vi "validateNewBalls.vi"(7 "timeToValidateBall":dbl=0.5, 8 "error in (no error)":errorcluster, 10 "array of cameras in":T1[](array[typedef]) {"robots_blue"."height" format="%+4.3f"; "robots_blue"."pixel_y" format="%+4.3f"; "robots_blue"."pixel_x" format="%+4.3f"; "robots_blue"."orientation" format="%+4.3f"; "robots_blue"."y" format="%+4.3f"; "robots_blue"."confidence" format="%4.3f"; "robots_blue"."x" format="%+4.3f"; "robots_yellow"."height" format="%+4.3f"; "robots_yellow"."pixel_y" format="%+4.3f"; "robots_yellow"."pixel_x" format="%+4.3f"; "robots_yellow"."orientation" format="%+4.3f"; "robots_yellow"."y" format="%+4.3f"; "robots_yellow"."confidence" format="%4.3f"; "robots_yellow"."x" format="%+4.3f"}, 11 "Vision in":refnum<class "Vision.lvclass">) -> (0 "error out":errorcluster, 2 "Array of cameras out":T1[](array[typedef]) {"robots_blue"."height" format="%+4.3f"; "robots_blue"."pixel_y" format="%+4.3f"; "robots_blue"."pixel_x" format="%+4.3f"; "robots_blue"."orientation" format="%+4.3f"; "robots_blue"."y" format="%+4.3f"; "robots_blue"."confidence" format="%4.3f"; "robots_blue"."x" format="%+4.3f"; "robots_yellow"."height" format="%+4.3f"; "robots_yellow"."pixel_y" format="%+4.3f"; "robots_yellow"."pixel_x" format="%+4.3f"; "robots_yellow"."orientation" format="%+4.3f"; "robots_yellow"."y" format="%+4.3f"; "robots_yellow"."confidence" format="%4.3f"; "robots_yellow"."x" format="%+4.3f"}, 3 "Vision out":refnum<class "Vision.lvclass">)   [LabVIEW 2022 SP3, in "Vision.lvclass"]
uses:
  Vision.lvclass
  Old vision/Controls/SSL Detection Frame.ctl
  Old vision/Controls/SSL Detection Robot.ctl
  <vilib>/Analysis/Matrix/Datatypes/RealMatrix.ctl
  Old vision/Controls/SSL Detection Ball.ctl
  newBallValidate.ctl
  <vilib>/Analysis/_algsub.llb/Real Vector Norm.vi
  <vilib>/Analysis/NI_AALPro.lvlib
  <vilib>/Analysis/Matrix/NI_Matrix.lvlib
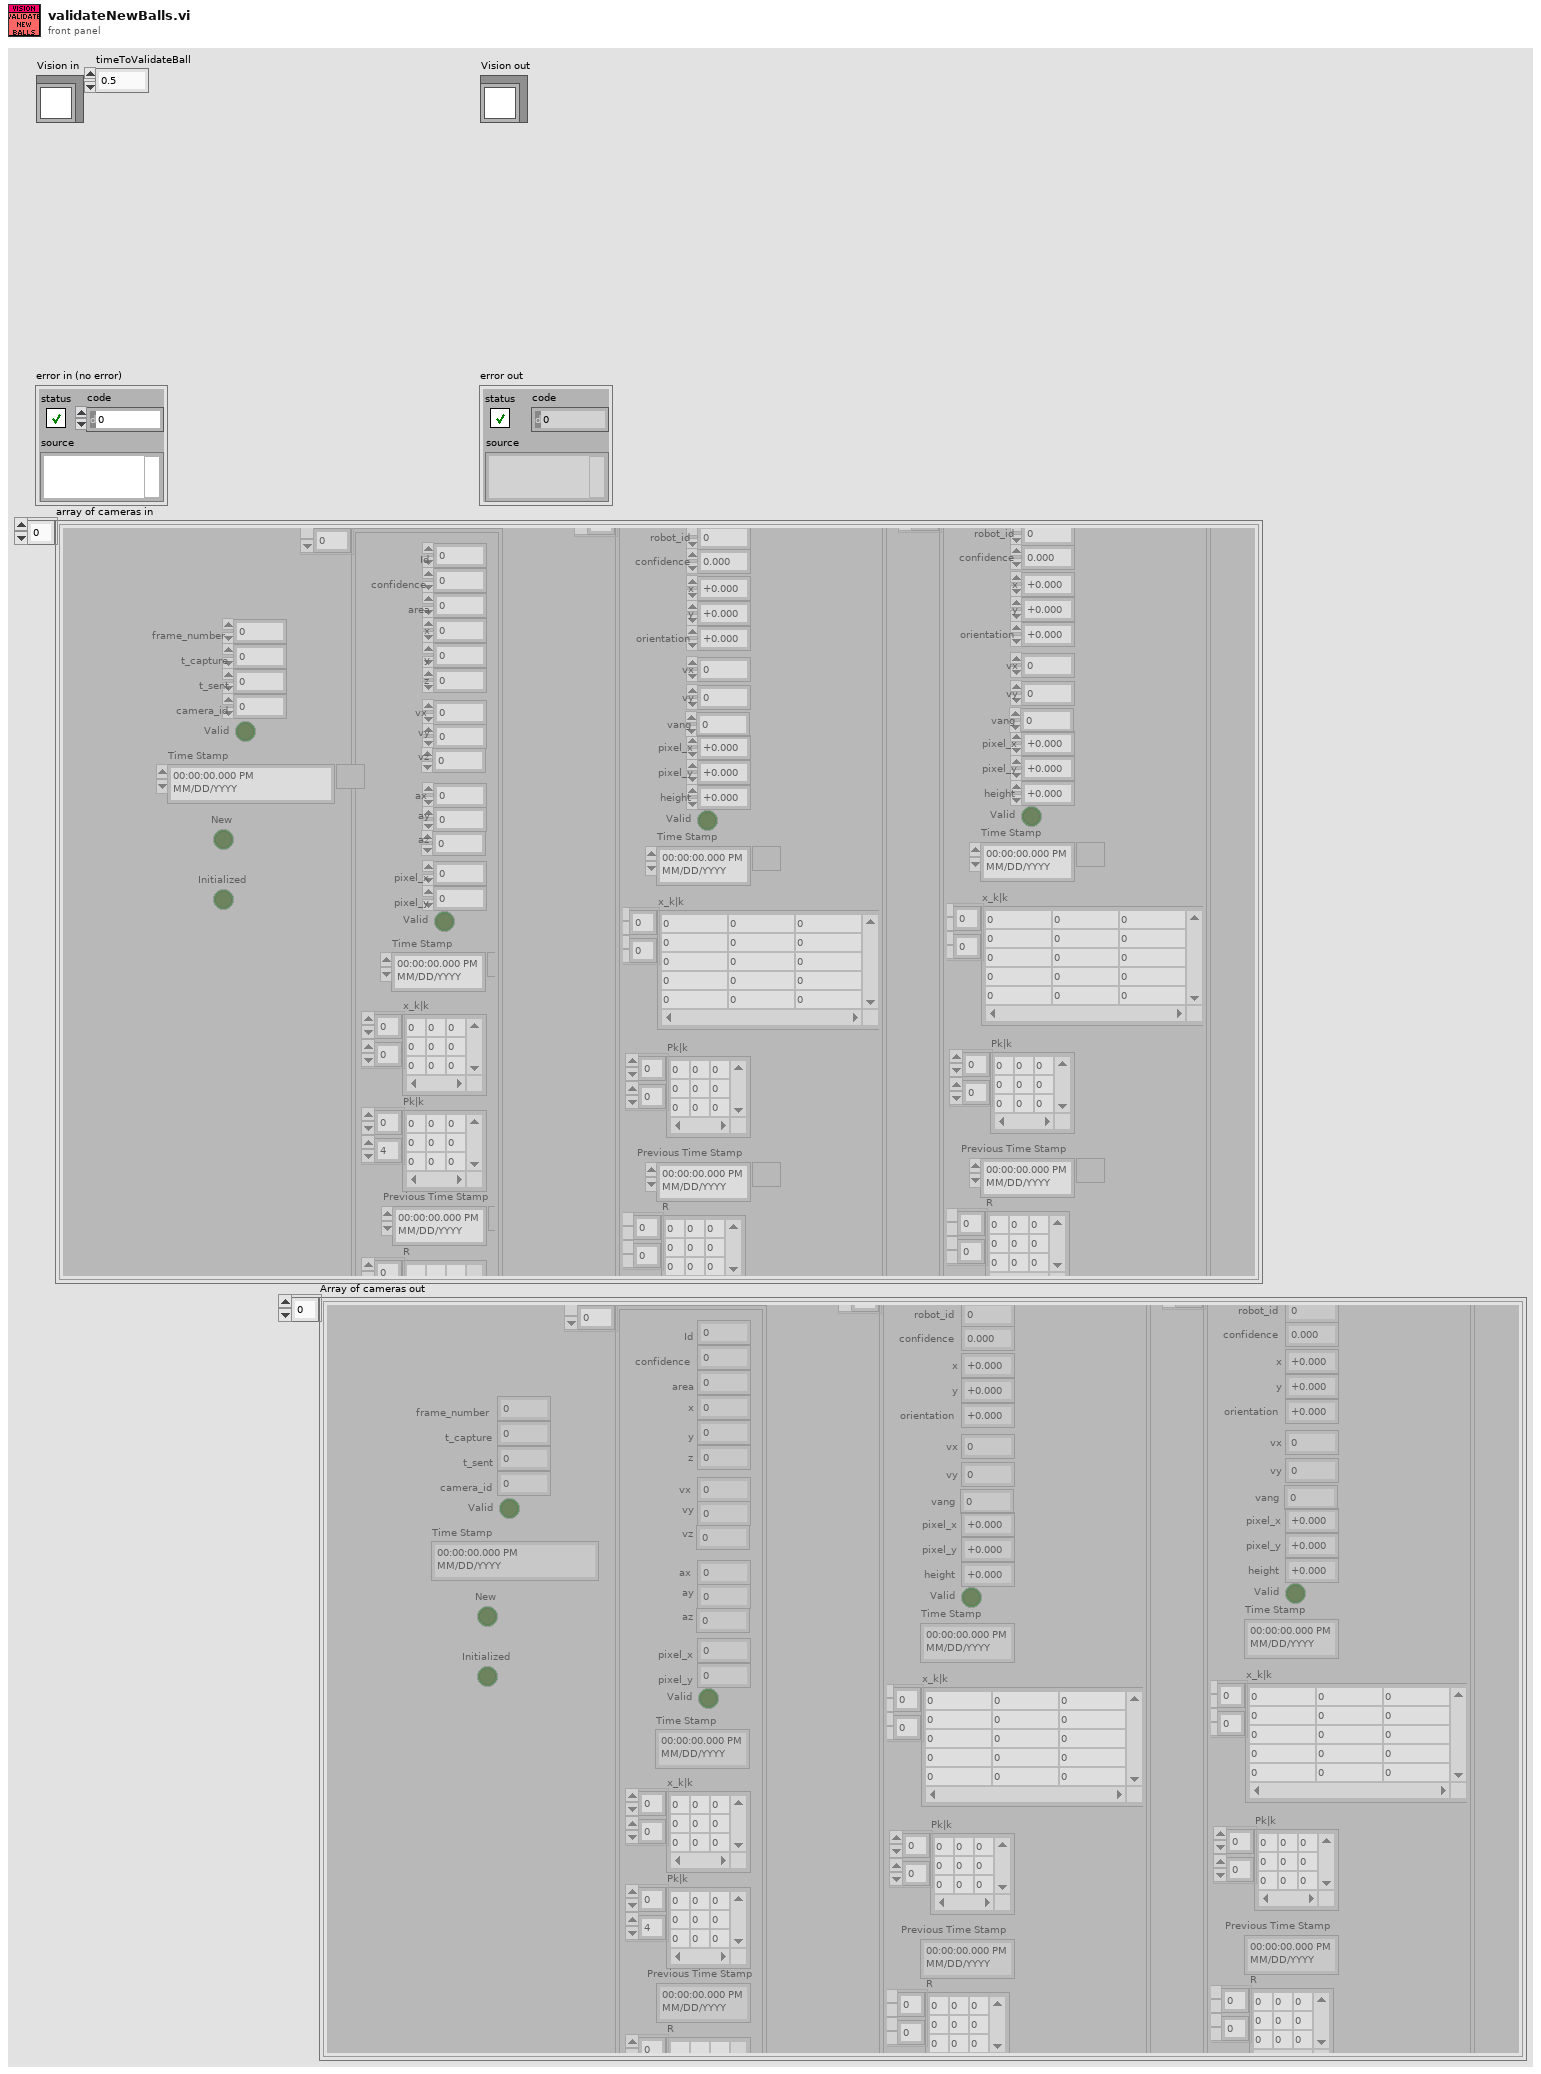
[diagram p1: front panel]
types:
  T1 = typedef "SSL Detection Frame.ctl" = cluster{"frame_number":u32, "t_capture":dbl, "t_sent":dbl, "camera_id":u32, "robots_yellow":T2[], "robots_blue":T2[], "balls":T4[], "Valid":bool, "Time Stamp":timestamp, "New":bool, "Initialized":bool}
  T2 = typedef "SSL Detection Robot.ctl" = cluster{"x":sgl, "robot_id":u32, "confidence":sgl, "y":sgl, "orientation":sgl, "pixel_x":sgl, "pixel_y":sgl, "height":sgl, "Valid":bool, "Time Stamp":timestamp, "x_k|k":T3, "Pk|k":T3, "Previous Time Stamp":timestamp, "R":T3, "vx":dbl, "vy":dbl, "vang":dbl}
  T3 = typedef "NI_Matrix.lvlib/RealMatrix.ctl" = dbl[][]
  T4 = typedef "SSL Detection Ball.ctl" = cluster{"x":sgl, "area":u32, "confidence":sgl, "y":sgl, "z":sgl, "pixel_x":sgl, "pixel_y":sgl, "Valid":bool, "Time Stamp":timestamp, "x_k|k":T3, "Pk|k":T3, "Id":u32, "Previous Time Stamp":timestamp, "R":T3, " vx":sgl, "vy":dbl, "vz":dbl, " ax":sgl, "ay":dbl, "az":dbl}
  T5 = typedef "newBallValidate.ctl" = cluster{"Ball_id":dbl, "camera_id":dbl, "BallPosition":dbl[], "timestamp":timestamp}
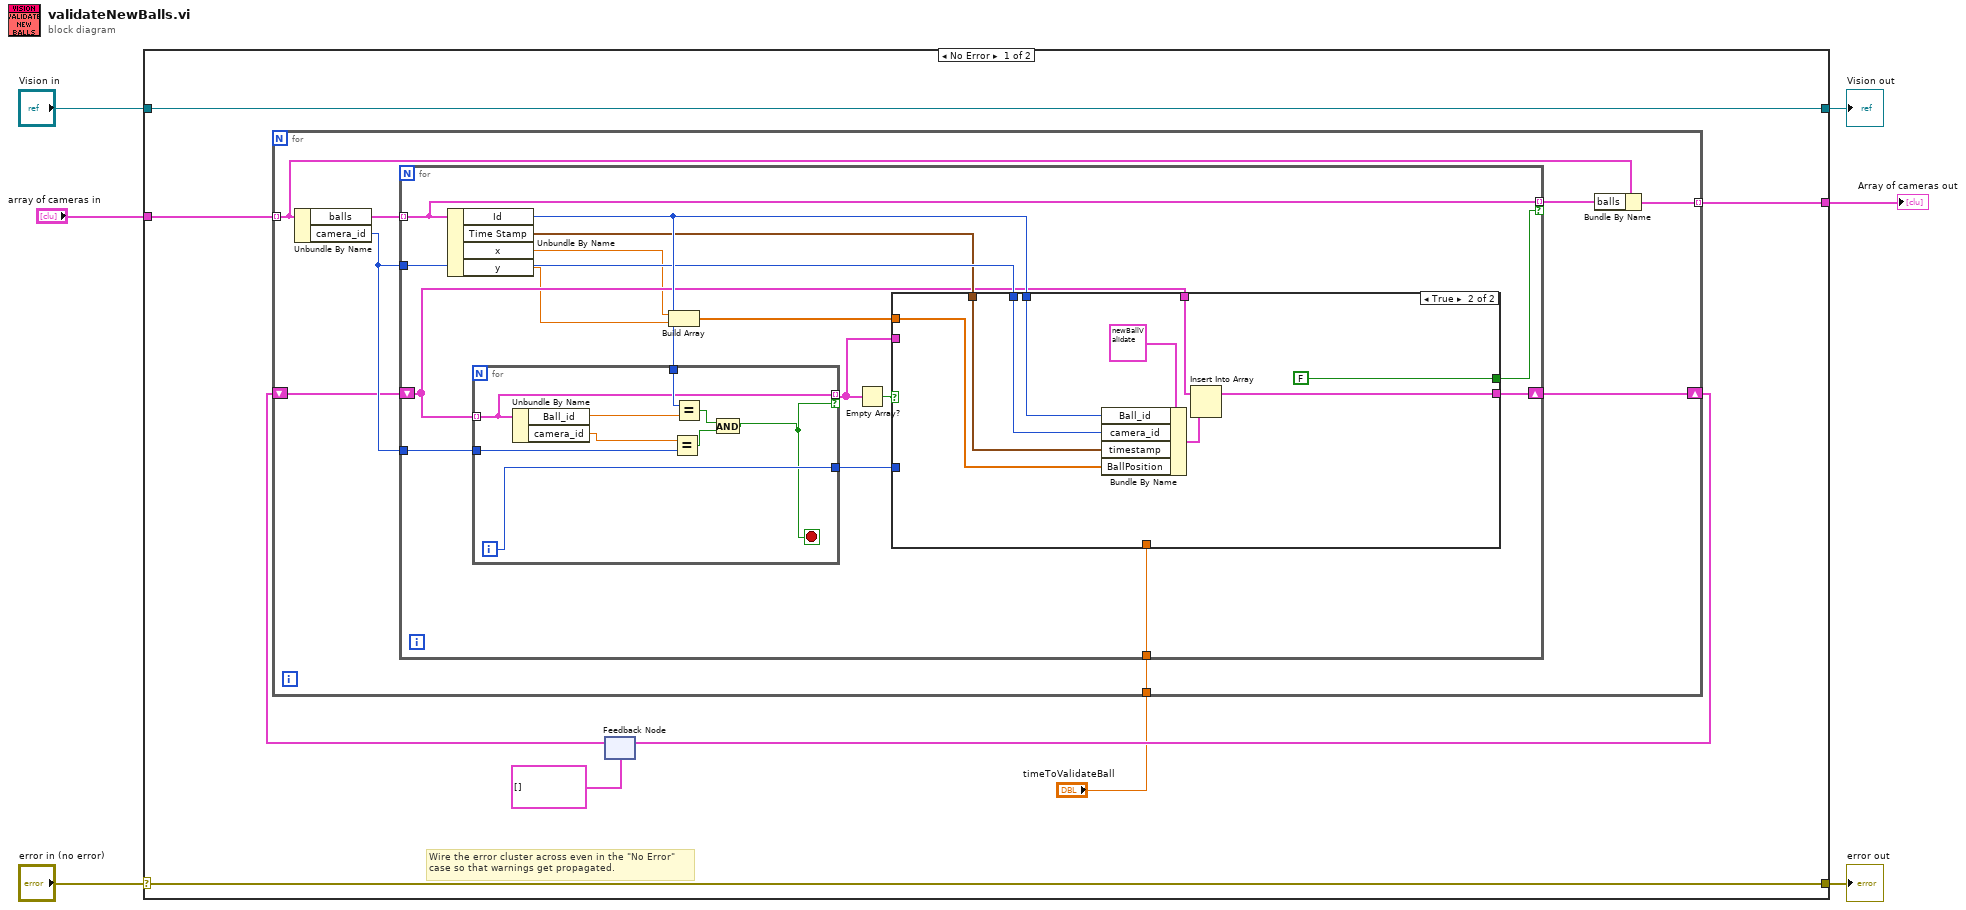
[diagram p0: block diagram]
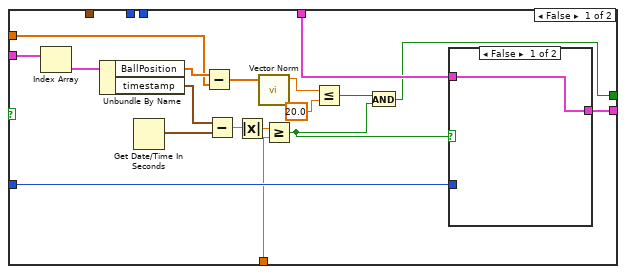
[diagram p2: hidden frame]
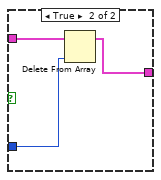
[diagram p3: hidden frame]
diagram:
  n1 = case shown="No Error" "error in (no error)" {
    selector: "error in (no error)" -> [w13 w79]
    tunnel: [w13 w79] -> w5
    tunnel: [w14 w78] -> w3
    tunnel: "Vision in" -> [w14 w78]
    tunnel: "array of cameras in" -> [w12 _]
    tunnel: [w8 _] -> w1
    frame No Error {
      # "Wire the error cluster across even in the \"No Error\"\ncase so that warnings get propagated."
      n2 = feedback #1(T5[] [] ("Array")) -> (w10:T5[])
      n3 = for {
        tunnel: w12 -> [w18] mode=indexing
        shift-right: [w20] -> w9
        shift-left: w10 -> [w19]
        tunnel: [w16] -> w8 mode=indexing
        tunnel: "timeToValidateBall" -> [w15]
        n4 = Unbundle By Name(w18) -> ("balls"=w22:T4[], "camera_id"=w21:u32)
        n5 = for {
          tunnel: w22 -> [w28] mode=indexing
          tunnel: w21 -> [w37]
          tunnel: w21 -> [w34]
          shift-right: [w32] -> w20
          shift-left: w19 -> [w31]
          tunnel: [w28] -> w17 mode=indexing if=w27
          tunnel: w15 -> [w23]
          n6 = Unbundle By Name(w28) -> ("Id"=w35:u32, "Time Stamp"=w33:timestamp, "x"=w24:sgl, "y"=w25:sgl)
          n7 = for {
            tunnel: w31 -> [w71] mode=indexing
            tunnel: w35 -> [w77]
            tunnel: w37 -> [w74]
            tunnel: [w71] -> w30 mode=indexing if=w69
            tunnel: [w70] -> w26
            i -> [w70]
            stop <- w69 stop-if-true
            n8 = Unbundle By Name(w71) -> ("Ball_id"=w76:dbl, "camera_id"=w75:dbl)
            n9 = Equal?(x=w75, y=w74) -> (x = y?=w72:bool)
            n10 = Equal?(x=w77, y=w76) -> (x = y?=w73:bool)
            n11 = And(x=w73, y=w72) -> (x .and. y?=w69:bool)
          }
          n12 = Build Array(w24, w25) -> (w29:sgl[])
          n13 = Empty Array?(array=w30) -> (empty?=w36:bool)
          n14 = case shown="True" w36 {
            tunnel: w31 -> [w47 w68]
            tunnel: w35 -> [_ w65]
            tunnel: w34 -> [_ w64]
            tunnel: w33 -> [_ w60]
            tunnel: [w48 w63] -> w32
            tunnel: w30 -> [w55 _]
            tunnel: w29 -> [w52 w62]
            tunnel: [w42 FALSE] -> w27
            tunnel: w26 -> [w46 _]
            tunnel: w23 -> [w38 _]
            frame False {
              n15 = Index Array(array=w55) -> (element=w54:T5)  [unwired: 1 in]
              n16 = Unbundle By Name(w54) -> ("BallPosition"=w53:dbl[], "timestamp"=w44:timestamp)
              n17 = Get Date/Time In Seconds() -> (seconds since 1Jan1904=w43:timestamp)
              n18 = Subtract(x=w53, y=w52) -> (x-y=w51:dbl[])
              n19 = Subtract(x=w44, y=w43) -> (x-y=w40:dbl)
              n20 = Absolute Value(x=w40) -> (abs(x)=w39:dbl)
              n21 = call-poly <vilib>:"Vector Norm.vi"("Input Vector"=w51) -> ("norm"=w50:dbl)  [unwired: 9 in, 1 out]
              n22 = Greater Or Equal?(x=w39, y=w38) -> (x >= y?=w41:bool)
              n23 = Less Or Equal?(x=w50, y=20.0) -> (x <= y?=w45:bool)
              n24 = And(x=w45, y=w41) -> (x .and. y?=w42:bool)
              n25 = case shown="False" w41 {
                tunnel: [w56 w57] -> w48
                tunnel: w47 -> [w56 w59]
                tunnel: w46 -> [_ w58]
                frame False {
                }
                frame True {
                  n26 = Delete From Array(array=w59, index=w58) -> (array with subset deleted=w57:T5[])  [unwired: 1 in, 1 out]
                }
              }
            }
            frame True {
              n27 = Bundle By Name(cluster=T5 {"Ball_id"=0.0, "camera_id"=0.0, "BallPosition"=[], "timestamp"=timestamp(0 s since 1904-01-01)} ("newBallsValidade 2"), "Ball_id"=w65, "camera_id"=w64, "timestamp"=w60, "BallPosition"=w62) -> (w66:T5)
              n28 = Insert Into Array(array=w68, new element=w66) -> (w63:T5[])  [unwired: 1 in]
            }
          }
        }
        n29 = Bundle By Name(cluster=w18, "balls"=w17) -> (w16:T1)
      }
      n30 = feedback-in #1(w9) -> ()
    }
    frame Error {
    }
  }
  "error out" <- w5
  "Vision out" <- w3
  "Array of cameras out" <- w1
